vi "Navigate and Wait.vi"(6 "Timeout (Inf)":i32=-1, 7 "html Source (URL)":bool, 8 "error in (no error)":errorcluster, 10 "Source":string, 11 "WebView2 Control in":refnum<class "WebView2 QControl.lvclass">) -> (0 "error out":errorcluster, 2 "Timed Out":bool, 3 "WebView2 Control out":refnum<class "WebView2 QControl.lvclass">)   [LabVIEW 2020, in "WebView2 QControl.lvlib" / "WebView2 QControl.lvclass"]
uses:
  WebView2 QControl.lvclass
  WebView2 QControl.lvclass/WebView2 QControl.ctl
  Webview2 Lib/WebView2 Control Object/WebView2 Control.lvclass
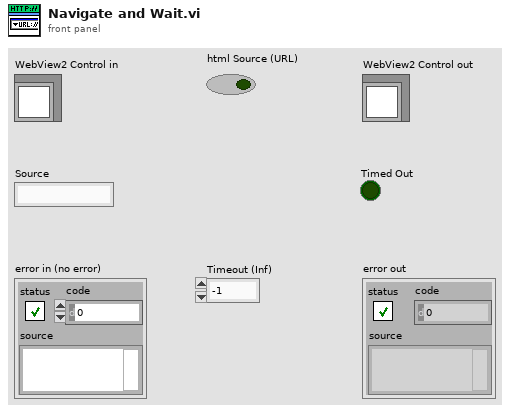
[diagram p1: front panel]
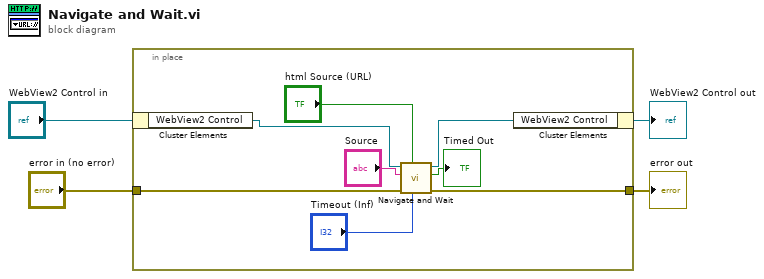
[diagram p0: block diagram]
diagram:
  n1 = in-place {
    in-place-border: "error in (no error)" -> [w12]
    in-place-border: [w11] -> w1
    n2 = in-place-cluster #1("WebView2 Control in") -> ("WebView2 Control"=w10:refnum<class "WebView2 Control.lvclass">)
    n3 = call "Navigate and Wait.vi"("Timeout (Inf)"="Timeout (Inf)", "html Source (URL)"="html Source (URL)", "error in (no error)"=w12, "Source"="Source", "WebView2 Control in"=w10) -> ("error out"=w11:errorcluster, "Timed Out"=→"Timed Out":bool, "WebView2 Control out"=w9:refnum<class "WebView2 Control.lvclass">)  [unwired: 4 in]
    n4 = in-place-cluster #1("WebView2 Control"=w9) -> (→"WebView2 Control out":refnum<class "WebView2 QControl.lvclass">)
  }
  "error out" <- w1
